vi "Get Hand Profit or Loss v2.vi"(10 "Dealt Player Name":string, 11 "Hand History String":string) -> (3 "Profit/Loss (BBs)":dbl)   [LabVIEW 2021]
uses:
  <vilib>/regexp/Match Regular Expression.xnode
panel:
  out "Big blind":dbl
  out "Profit/Loss":dbl
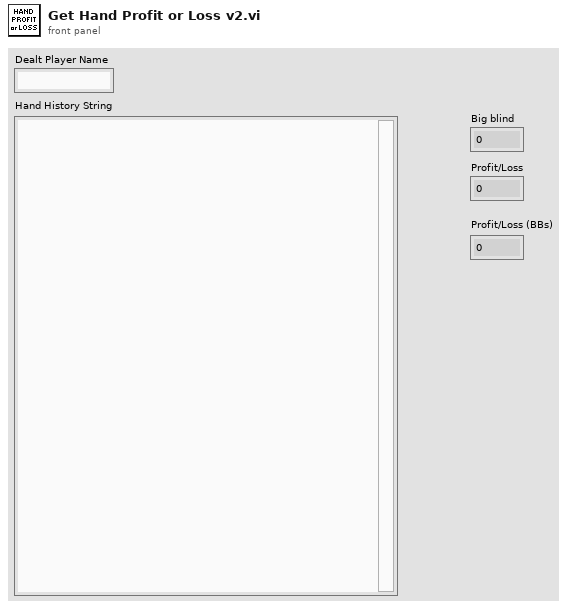
[diagram p1: front panel]
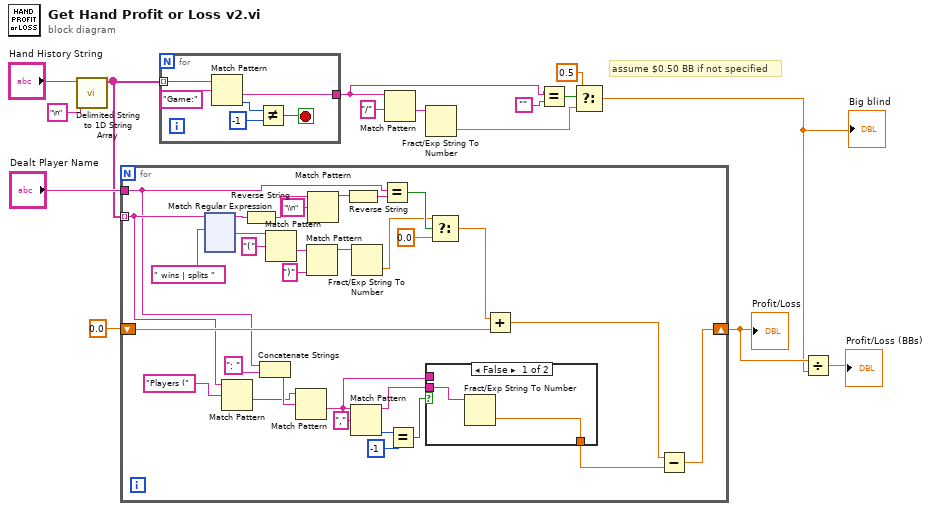
[diagram p0: block diagram]
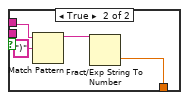
[diagram p2: hidden frame]
diagram:
  # "assume $0.50 BB if not specified"
  n1 = call <vilib>:"Delimited String to 1D String Array.vi"("delimiter"="\n", "delimited string"="Hand History String") -> ("string array"=w7:string[])  [unwired: 9 in]
  n2 = for {
    tunnel: w7 -> [w20] mode=indexing
    tunnel: "Dealt Player Name" -> [w19]
    shift-right: [w16] -> w9
    shift-left: 0.0 -> [w32]
    n3 = xnode "Match Regular Expression"("input string"=w20, "regular expression"=" wins | splits ") -> ("before match"=w37:string, "after match"=w36:string)  [unwired: 4 in, 3 out]
    n4 = Match Pattern(string=w20, regular expression="Players (") -> (after substring=w27:string)  [unwired: 1 in, 3 out]
    n5 = Reverse String(1:w37) -> (0:w42:string)
    n6 = Concatenate Strings(w19, ": " ("string")) -> (w28:string)
    n7 = Match Pattern(string=w36, regular expression="(") -> (after substring=w40:string)  [unwired: 1 in, 3 out]
    n8 = Match Pattern(string=w27, regular expression=w28) -> (after substring=w18:string)  [unwired: 1 in, 3 out]
    n9 = Match Pattern(string=w40, regular expression=")") -> (before substring=w38:string)  [unwired: 1 in, 3 out]
    n10 = Match Pattern(string=w42, regular expression="\\n") -> (before substring=w44:string)  [unwired: 1 in, 3 out]
    n11 = Reverse String(1:w44) -> (0:w43:string)
    n12 = Match Pattern(string=w18, regular expression=",") -> (before substring=w22:string, offset past match=w25:i32)  [unwired: 1 in, 2 out]
    n13 = Fract/Exp String To Number(string=w38) -> (number=w34:dbl)  [unwired: 3 in, 1 out]
    n14 = Equal?(x=w19, y=w43) -> (x = y?=w35:bool)
    n15 = Equal?(x=w25, y=-1) -> (x = y?=w23:bool)
    n16 = case shown="False" w23 {
      tunnel: w22 -> [w48 _]
      tunnel: [w47 w49] -> w21
      tunnel: w18 -> [_ w52]
      frame False {
        n17 = Fract/Exp String To Number(string=w48) -> (number=w47:dbl)  [unwired: 3 in, 1 out]
      }
      frame True {
        n18 = Match Pattern(string=w52, regular expression=")") -> (before substring=w50:string)  [unwired: 1 in, 3 out]
        n19 = Fract/Exp String To Number(string=w50) -> (number=w49:dbl)  [unwired: 3 in, 1 out]
      }
    }
    n20 = Select(t=w34, s=w35, f=0.0) -> (s? t:f=w31:dbl)
    n21 = Add(x=w31, y=w32) -> (x+y=w17:dbl)
    n22 = Subtract(x=w17, y=w21) -> (x-y=w16:dbl)
  }
  "Profit/Loss" <- w9
  n23 = for {
    tunnel: w7 -> [w175] mode=indexing
    tunnel: [w170] -> w4
    stop <- w171 stop-if-true
    n24 = Match Pattern(string=w175, regular expression="Game:") -> (after substring=w170:string, offset past match=w173:i32)  [unwired: 1 in, 2 out]
    n25 = Not Equal?(x=w173, y=-1) -> (x != y?=w171:bool)
  }
  n26 = Match Pattern(string=w4, regular expression="/") -> (after substring=w12:string)  [unwired: 1 in, 3 out]
  n27 = Fract/Exp String To Number(string=w12) -> (number=w2:dbl)  [unwired: 3 in, 1 out]
  n28 = Equal?(x=w4, y="") -> (x = y?=w6:bool)
  n29 = Select(t=0.5, s=w6, f=w2) -> (s? t:f=w1:dbl)
  "Big blind" <- w1
  n30 = Divide(x=w9, y=w1) -> (x/y=→"Profit/Loss (BBs)":dbl)
